vi "After Launch Init.vi"(8 "error in (no error)":errorcluster, 11 "CS++DMM in":refnum<class "CS++DMM.lvclass">) -> (0 "error out":errorcluster, 3 "CS++DMM out":refnum<class "CS++DMM.lvclass">)   [LabVIEW 2013, in "CS++DMM.lvlib" / "CS++DMM.lvclass"]
doc: "Use <b>Pre Launch init.vi</b> method for sanity checks that are supposed to prevent the actor from launching if they fail. Use <B>this</B> method instead to initialize this actor when it has been activated. A corresponding high priority message will become dispatched before the <B>Actor Core.vi</b> is called.\n\nRefer also to the ongoing discussion at https://decibel.ni.com/content/message/57394#57394."
uses:
  CS++DMM.lvclass
  Core/Classes/CS++ProcessVariables/SVConnection/SVConnection.lvclass
  CS++DMM.lvclass/CS++DMM.ctl
  Core/Classes/CS++ProcessVariables/PVConnection/PVConnection.lvclass/PVConnection.ctl
  Core/Actors/CS++DeviceActor/CS++DeviceActor.lvclass
  Core/Actors/CS++DeviceActor/CS++DeviceActor.lvclass/CS++DeviceActor.ctl
  <vilib>/ActorFramework/Actor/Actor.lvclass/Actor.ctl
  <vilib>/ActorFramework/Message Enqueuer/Message Enqueuer.lvclass/Message Enqueuer.ctl
  CS++DMM Messages/Read Single-Point Msg/Read Single-Point Msg.lvclass
  CS++DMM Messages/Read Single-Point Msg/Read Single-Point Msg.lvclass/Read Single-Point Msg.ctl
  CS++DMM Messages/Read Single-Point Msg/Write maximum time.vi
  <vilib>/ActorFramework/Message Enqueuer/Init from Existing Queue.vi
  <vilib>/ActorFramework/Message Enqueuer/Message Enqueuer.lvclass
  Core/Classes/CS++ProcessVariables/PVConnection/PVConnection.lvclass
  <vilib>/ActorFramework/Actor/Actor.lvclass
  CS++DMM Messages/Read Multi-Point [MP] Msg/Read Multi-Point [MP] Msg.lvclass
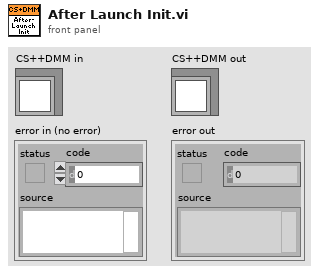
[diagram p1: front panel]
types:
  T1 = cluster{"Write Access":enum8{"Allowed", "Required", "None"}, "Read Access":enum8{"Allowed", "Required", "None"}}
  T2 = cluster{"Reading":string, "MPReading":string, "IsOverRange":string, "MeasurementFunction":string, "AbsoluteResolution":string, "Range":string, "ApertureTime":string, "ApertureTimeUnit":string, "ActualRange":string, "SampleInterval":string, "TriggerCount":string, "SampleCount":string, "SampleTrigger":string, "MeasCompleteDest":string, "AutoZeroMode":string, "PowerLineFrequency":string, "FrequencyVoltageRange":string, "ACMinFrequency":string, "ACMaxFrequency":string, "TransducerType":string, "ThermocoupleType":string, "ReferenceJunctionType":string, "FixedReferenceJunction":string, "Alpha":string, "Resistance":string, "TriggerSource":string, "TriggerDelay":string, "TriggerSlope":string}
  T3 = cluster{"[0]":refnum<class "SVConnection.lvclass">, "[1]":refnum<class "SVConnection.lvclass">, "[2]":refnum<class "SVConnection.lvclass">, "[3]":refnum<class "SVConnection.lvclass">, "[4]":refnum<class "SVConnection.lvclass">, "[5]":refnum<class "SVConnection.lvclass">, "[6]":refnum<class "SVConnection.lvclass">, "[7]":refnum<class "SVConnection.lvclass">, "[8]":refnum<class "SVConnection.lvclass">, "[9]":refnum<class "SVConnection.lvclass">, "[10]":refnum<class "SVConnection.lvclass">, "[11]":refnum<class "SVConnection.lvclass">, "[12]":refnum<class "SVConnection.lvclass">, "[13]":refnum<class "SVConnection.lvclass">, "[14]":refnum<class "SVConnection.lvclass">, "[15]":refnum<class "SVConnection.lvclass">, "[16]":refnum<class "SVConnection.lvclass">, "[17]":refnum<class "SVConnection.lvclass">, "[18]":refnum<class "SVConnection.lvclass">, "[19]":refnum<class "SVConnection.lvclass">, "[20]":refnum<class "SVConnection.lvclass">, "[21]":refnum<class "SVConnection.lvclass">, "[22]":refnum<class "SVConnection.lvclass">, "[23]":refnum<class "SVConnection.lvclass">, "[24]":refnum<class "SVConnection.lvclass">, "[25]":refnum<class "SVConnection.lvclass">, "[26]":refnum<class "SVConnection.lvclass">, "[27]":refnum<class "SVConnection.lvclass">}
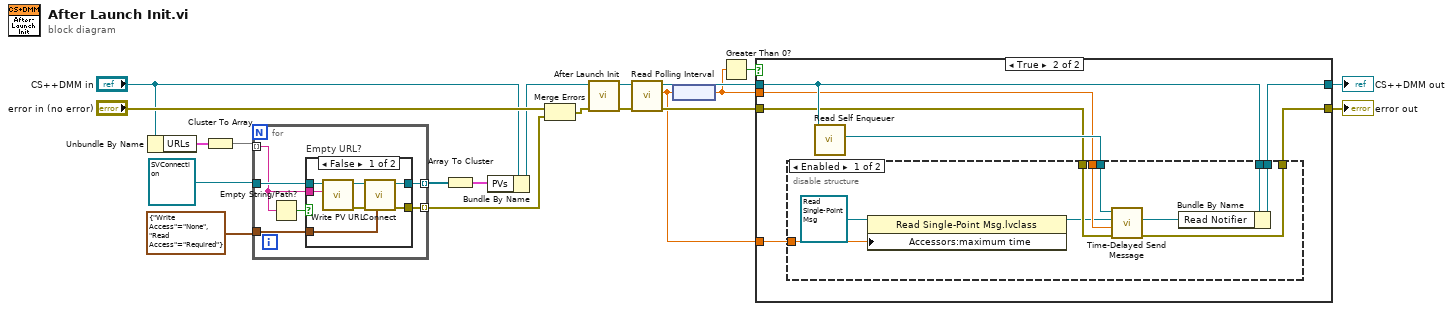
[diagram p0: block diagram]
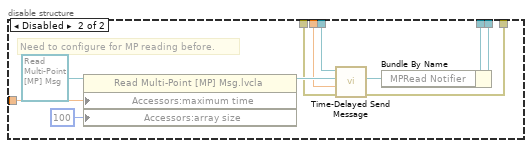
[diagram p3: hidden frame]
diagram:
  n1 = Unbundle By Name("CS++DMM in") -> ("URLs"=w16:T2)
  n2 = Cluster To Array(cluster=w16) -> (array=w17:string[])
  n3 = for {
    tunnel: w17 -> [w22] mode=indexing
    tunnel: refnum<class "SVConnection.lvclass"> refnum ("CS++ProcessVariables.lvlib:SVConnection.lvclass") -> [w26]
    tunnel: T1 {"Write Access"=enum."None", "Read Access"=enum."Required"} ("Access") -> [w25]
    tunnel: [w24] -> w15 mode=indexing
    tunnel: [w21] -> w10 mode=indexing
    n4 = Empty String/Path?(string/path=w22) -> (empty?=w23:bool)
    n5 = case "Empty URL?" shown="False" w23 {
      tunnel: w26 -> [w33 w34]
      tunnel: w22 -> [w32 _]
      tunnel: w25 -> [w29 _]
      tunnel: [w28 w34] -> w24
      tunnel: [w27 _] -> w21
      frame False {
        n6 = call "Write PV URL.vi"("PV URL"=w32, "PVConnection in"=w33) -> ("error out"=w30:errorcluster, "PVConnection out"=w31:refnum<class "SVConnection.lvclass">)  [unwired: 8 in]
        n7 = call-dynamic "Connect.vi"("Access"=w29, "error in (no error)"=w30, "PVConnection in"=w31) -> ("error out"=w27:errorcluster, "PVConnection out"=w28:refnum<class "SVConnection.lvclass">)  [unwired: 7 in]
      }
      frame True {
      }
    }
  }
  n8 = Array To Cluster(array=w15) -> (cluster=w14:T3)
  n9 = Bundle By Name(cluster="CS++DMM in", "PVs"=w14) -> (w12:refnum<class "CS++DMM.lvclass">)
  n10 = Merge Errors("error in (no error)", w10) -> (w11:errorcluster)
  n11 = call-parent "After Launch Init.vi"("error in (no error)"=w11, "CS++DeviceActor in"=w12) -> ("error out"=w5:errorcluster, "CS++DeviceActor out"=w7:refnum<class "CS++DMM.lvclass">)  [unwired: 8 in]
  n12 = call "Read Polling Interval.vi"("error in (no error)"=w5, "CS++DeviceActor in"=w7) -> ("error out"=w4:errorcluster, "Polling Interval"=w1:dbl[unit], "CS++DeviceActor out"=w6:refnum<class "CS++DMM.lvclass">)  [unwired: 7 in]
  n13 = node(w1) -> (w3:dbl)
  n14 = Greater Than 0?(x=w3) -> (x > 0?=w2:bool)
  n15 = case shown="True" w2 {
    tunnel: [w36 w43] -> w9
    tunnel: [w35 w37] -> w8
    tunnel: w6 -> [w36 w42]
    tunnel: w4 -> [w35 w40]
    tunnel: w3 -> [_ w39]
    tunnel: w1 -> [_ w38]
    frame False {
    }
    frame True {
      n16 = call <vilib>:"Read Self Enqueuer.vi"("Actor"=w42) -> ("Self Enqueuer"=w41:refnum<class "Message Enqueuer.lvclass">)  [unwired: 10 in]
      n17 = disable-structure shown="Enabled" {
        disable-tunnel: [w53 w56] -> w43
        disable-tunnel: w42 -> [w52 w57]
        disable-tunnel: w41 -> [w50 w60]
        disable-tunnel: w40 -> [w49 w58]
        disable-tunnel: w39 -> [w48 w59]
        disable-tunnel: w38 -> [w45 w61]
        disable-tunnel: [w44 w54] -> w37
        frame Enabled {
          n18 = property class="Read Single-Point Msg.lvclass"(reference=refnum<class "Read Single-Point Msg.lvclass"> refnum ("CS++DMM.lvlib:Read Single-Point Msg.lvclass"), "Accessors:maximum time"=w45) -> (reference out=w46:refnum<class "Read Single-Point Msg.lvclass">)  [unwired: 1 in, 1 out]
          n19 = call <vilib>:"Time-Delayed Send Message.vi"("error in (no error)"=w49, "Milliseconds To Wait"=w48, "Message"=w46, "Message Enqueuer"=w50) -> ("error out"=w44:errorcluster, "Delivery Notifier"=w51:refnum<notifier>)  [unwired: 6 in]
          n20 = Bundle By Name(cluster=w52, "Read Notifier"=w51) -> (w53:refnum<class "CS++DMM.lvclass">)
        }
        frame Disabled {
          # "Need to configure for MP reading before."
          n21 = property class="Read Multi-Point [MP] Msg.lvcla"(reference=refnum<class "Read Multi-Point [MP] Msg.lvclass"> refnum ("CS++DMM.lvlib:Read Multi-Point [MP] Msg.lvclass"), "Accessors:maximum time"=w61, "Accessors:array size"=100 ("array size")) -> (reference out=w63:refnum<class "Read Multi-Point [MP] Msg.lvclass">)  [unwired: 1 in, 1 out]
          n22 = call <vilib>:"Time-Delayed Send Message.vi"("error in (no error)"=w58, "Milliseconds To Wait"=w59, "Message"=w63, "Message Enqueuer"=w60) -> ("error out"=w54:errorcluster, "Delivery Notifier"=w55:refnum<notifier>)  [unwired: 6 in]
          n23 = Bundle By Name(cluster=w57, "MPRead Notifier"=w55) -> (w56:refnum<class "CS++DMM.lvclass">)
        }
      }
    }
  }
  "error out" <- w8
  "CS++DMM out" <- w9
